vi "Fit VI window to Panel Center.vi"(4 "Error In":errorcluster, 6 "Panel Ref":refnum<vi>, 7 "VI Ref (calling VI)":refnum<vi>) -> (0 "Error Out":errorcluster, 3 "dup VI Ref":refnum<vi>)   [LabVIEW 2017]
doc: "This VI is designed to center a callee VI's window in a caller VI's window.\n\nAuthored by Brandon Steele\nsupport@mooregoodideas.com\nwww.mooregoodideas.com\n\nCopyright (c) 2010, Moore Good Ideas, Inc.\n\nAll rights reserved.\n\nRedistribution and use in source and binary forms, with or without modification, are permitted provided that the following conditions are met:\n\n * Redistributions of source code must retain the above copyright notice, this list of conditions and the following disclaimer.\n * Redistributions in binary form must reproduce the above copyright notice, this list of conditions and the following disclaimer in the documentation and/or other materials provided with the distribution.\n * Neither the name of Moore Good Ideas, Inc. nor the names of its contributors may be used to endorse or promote products derived from this software without specific prior written permission.\n\nTHIS SOFTWARE IS PROVIDED BY THE COPYRIGHT HOLDERS AND CONTRIBUTORS \"AS IS\" AND ANY EXPRESS OR IMPLIED WARRANTIES, INCLUDING, BUT NOT LIMITED TO, THE IMPLIED WARRANTIES OF MERCHANTABILITY AND FITNESS FOR A PARTICULAR PURPOSE ARE DISCLAIMED. IN NO EVENT SHALL THE COPYRIGHT OWNER OR CONTRIBUTORS BE LIABLE FOR ANY DIRECT, INDIRECT, INCIDENTAL, SPECIAL, EXEMPLARY, OR CONSEQUENTIAL DAMAGES (INCLUDING, BUT NOT LIMITED TO, PROCUREMENT OF SUBSTITUTE GOODS OR SERVICES; LOSS OF USE, DATA, OR PROFITS; OR BUSINESS INTERRUPTION) HOWEVER CAUSED AND ON ANY THEORY OF LIABILITY, WHETHER IN CONTRACT, STRICT LIABILITY, OR TORT (INCLUDING NEGLIGENCE OR OTHERWISE) ARISING IN ANY WAY OUT OF THE USE OF THIS SOFTWARE, EVEN IF ADVISED OF THE POSSIBILITY OF SUCH DAMAGE."
panel:
  in  "Pane Ref":refnum<vi>
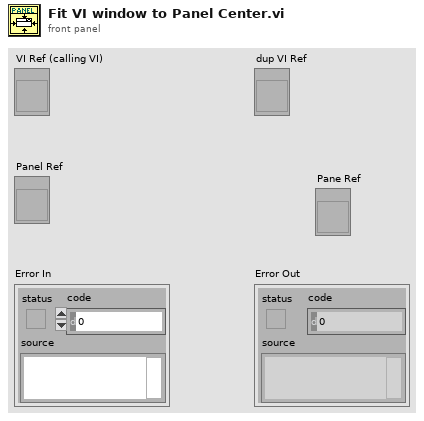
[diagram p1: front panel]
types:
  T1 = typedef "LVRectTypeDef.ctl" = cluster{"Left":i16, "Top":i16, "Right":i16, "Bottom":i16}
  T2 = cluster{"left":i16, "top":i16, "right":i16, "bottom":i16}
  T3 = typedef "LVAllMonitorsDisplayTypeDef.ctl" = cluster{"Bounds":cluster{"Left":i16, "Top":i16, "Right":i16, "Bottom":i16}, "Depth":i16}[]
  T4 = cluster{"Left":i16, "Top":i16, "Right":i16, "Bottom":i16}
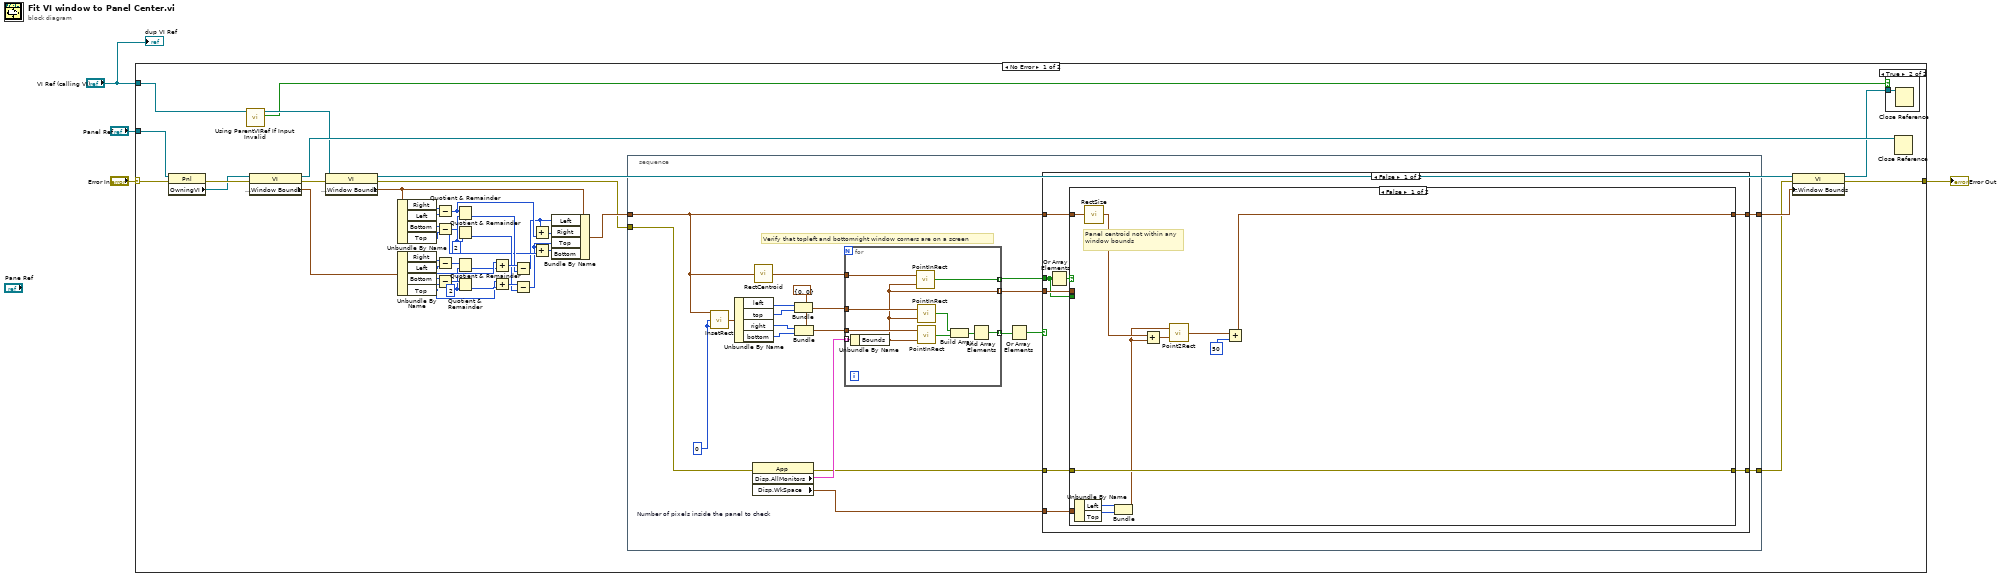
[diagram p0: block diagram]
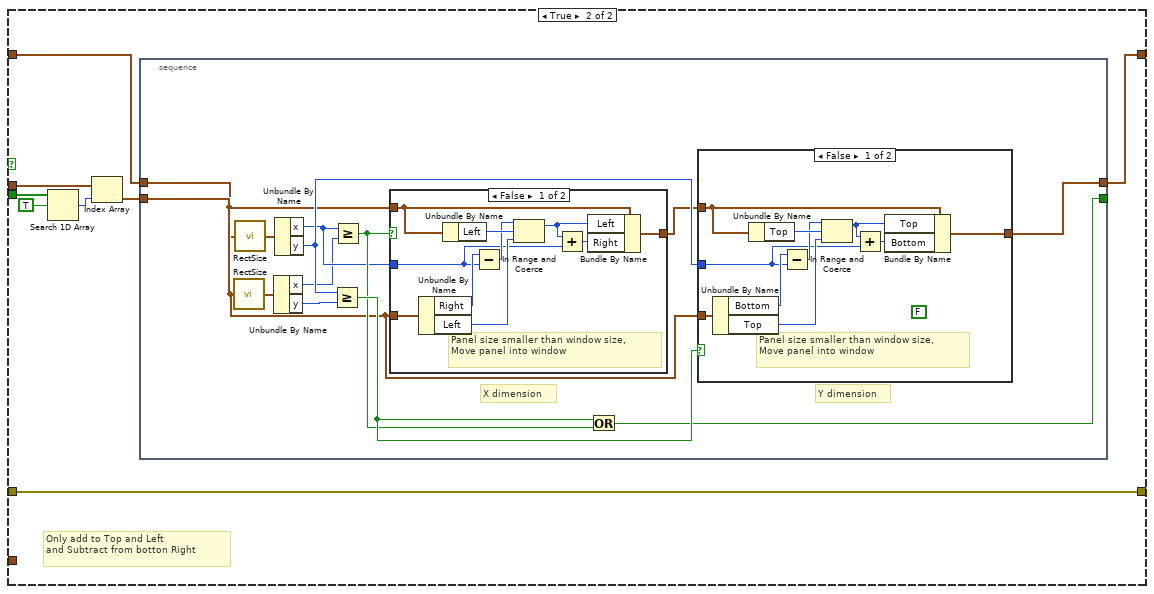
[diagram p2: hidden frame]
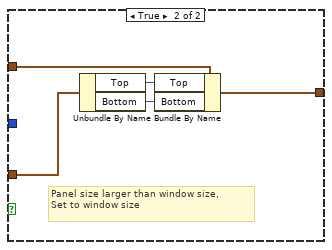
[diagram p3: hidden frame]
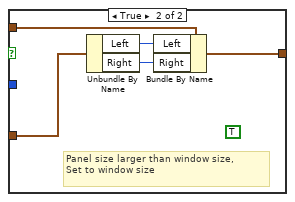
[diagram p4: hidden frame]
diagram:
  n1 = case shown="No Error" "Error In" {
    selector: "Error In" -> [w8 w151]
    tunnel: [w46 w151] -> w4
    tunnel: "Panel Ref" -> [w5 _]
    tunnel: "VI Ref (calling VI)" -> [w22 _]
    frame No Error {
      w39 = i16 2 ("y")
      w23 = i16 2 ("y")
      n2 = property class="Pnl"(reference=w5, error in=w8) -> (error out=w7:errorcluster, "OwningVI"=w6:refnum<vi>)  [unwired: 1 out]
      n3 = call "Using ParentVIRef If Input Invalid.vi"("VI Ref (calling VI)"=w22) -> ("Using Parent Ref(Need to Destroy)"=w11:bool, "VI Ref"=w19:refnum<vi>)  [unwired: 5 in]
      n4 = property class="VI"(reference=w6, error in=w7) -> (reference out=w21:refnum<vi>, error out=w40:errorcluster, "Front Panel Window:Window Bounds"=w45:T1)
      n5 = property class="VI"(reference=w19, error in=w40) -> (reference out=w26:refnum<vi>, error out=w10:errorcluster, "Front Panel Window:Window Bounds"=w14:T1)
      n6 = Unbundle By Name(w14) -> ("Right"=w35:i16, "Left"=w36:i16, "Bottom"=w37:i16, "Top"=w38:i16)
      n7 = Unbundle By Name(w45) -> ("Right"=w44:i16, "Left"=w34:i16, "Bottom"=w43:i16, "Top"=w31:i16)
      n8 = Subtract(x=w35, y=w36) -> (x-y=w25:i16)
      n9 = Subtract(x=w37, y=w38) -> (x-y=w24:i16)
      n10 = Subtract(x=w44, y=w34) -> (x-y=w42:i16)
      n11 = Subtract(x=w43, y=w31) -> (x-y=w41:i16)
      n12 = Quotient & Remainder(x=w25, y=w39) -> (floor(x/y)=w29:i16)  [unwired: 1 out]
      n13 = Quotient & Remainder(x=w24, y=w39) -> (floor(x/y)=w27:i16)  [unwired: 1 out]
      n14 = Quotient & Remainder(x=w42, y=w23) -> (floor(x/y)=w33:i16)  [unwired: 1 out]
      n15 = Quotient & Remainder(x=w41, y=w23) -> (floor(x/y)=w32:i16)  [unwired: 1 out]
      n16 = Add(x=w34, y=w33) -> (x+y=w30:i16)
      n17 = Add(x=w31, y=w32) -> (x+y=w28:i16)
      n18 = Subtract(x=w30, y=w29) -> (x-y=w17:i16)
      n19 = Subtract(x=w28, y=w27) -> (x-y=w16:i16)
      n20 = Add(x=w17, y=w25) -> (x+y=w15:i16)
      n21 = Add(x=w16, y=w24) -> (x+y=w18:i16)
      n22 = Bundle By Name(cluster=w14, "Left"=w17, "Right"=w15, "Top"=w16, "Bottom"=w18) -> (w13:T1)
      n23 = stacked-sequence {
        tunnel: [w57] -> w9
        tunnel: [w48] -> w12
        tunnel: w10 -> [w50]
        tunnel: w13 -> [w64]
        frame #0 {
          w59 = i16 0  # Number of pixels inside the panel to check
          w63 = cluster{"x":i16, "y":i16} {"x"=0, "y"=0} ("point")
          # "Verify that topleft and bottomright window corners are on a screen"
          n24 = call <vilib>:"InsetRect.vi"("dv"=w59, "dh"=w59, "rect"=w64) -> ("inset rect"=w53:T2)
          n25 = Unbundle By Name(w53) -> ("left"=w51:i16, "top"=w52:i16, "right"=w60:i16, "bottom"=w61:i16)
          n26 = property class="App"(error in=w50) -> (error out=w47:errorcluster, "Disp.AllMonitors"=w49:T3, "Disp.WkSpace"=w58:T1)  [unwired: 1 in, 1 out]
          n27 = call <vilib>:"RectCentroid.vi"("rect"=w64) -> ("point"=w65:cluster{"x":i16, "y":i16})
          n28 = Bundle(cluster=w63, "x"=w51, "y"=w52) -> (w54:cluster{"x":i16, "y":i16})
          n29 = Bundle(cluster=w63, "x"=w60, "y"=w61) -> (w62:cluster{"x":i16, "y":i16})
          n30 = for {
            tunnel: w49 -> [w149] mode=indexing
            tunnel: w54 -> [w148]
            tunnel: [w144] -> w55 mode=indexing
            tunnel: w62 -> [w143]
            tunnel: w65 -> [w142]
            tunnel: [w141] -> w66 mode=indexing
            tunnel: [w140] -> w67 mode=indexing
            n31 = Unbundle By Name(w149) -> ("Bounds"=w140:T4)
            n32 = call <vilib>:"PointInRect.vi"("rect"=w140, "point"=w142) -> ("pt in rect"=w141:bool)
            n33 = call <vilib>:"PointInRect.vi"("rect"=w140, "point"=w148) -> ("pt in rect"=w147:bool)
            n34 = call <vilib>:"PointInRect.vi"("rect"=w140, "point"=w143) -> ("pt in rect"=w146:bool)
            n35 = Build Array(w147, w146) -> (w145:bool[])
            n36 = And Array Elements(Boolean array=w145) -> (logical AND=w144:bool)
          }
          n37 = Or Array Elements(Boolean array=w55) -> (logical OR=w56:bool)
          n38 = case shown="False" w56 {
            tunnel: w47 -> [w70 w139]
            tunnel: [w69 w139] -> w57
            tunnel: w64 -> [w74 w138]
            tunnel: [w73 w138] -> w48
            tunnel: w58 -> [w75 _]
            tunnel: w66 -> [w68 _]
            tunnel: w67 -> [w71 _]
            frame False {
              n39 = Or Array Elements(Boolean array=w68) -> (logical OR=w72:bool)
              n40 = case shown="False" w72 {
                tunnel: w75 -> [w86 _]
                tunnel: w74 -> [w82 w89]
                tunnel: [w80 w87] -> w73
                tunnel: w71 -> [_ w91]
                tunnel: w70 -> [w79 w94]
                tunnel: [w79 w94] -> w69
                tunnel: w68 -> [_ w93]
                frame False {
                  # "Panel centroid not within any\nwindow bounds"
                  n41 = Unbundle By Name(w86) -> ("Left"=w85:i16, "Top"=w84:i16)
                  n42 = call <vilib>:"RectSize.vi"("rect"=w82) -> ("point"=w78:cluster{"x":i16, "y":i16})
                  n43 = Bundle("Left"=w85, "Top"=w84) -> (w76:cluster{"Left":i16, "Top":i16})  [unwired: 1 in]
                  n44 = Add(x=w78, y=w76) -> (x+y=w77:cluster{i16, i16})
                  n45 = call <vilib>:"Point2Rect.vi"("point b"=w77, "point a"=w76) -> ("rect"=w81:T2)
                  n46 = Add(x=w81, y=i16 50) -> (x+y=w80:T2)
                }
                frame True {
                  # "Only add to Top and Left\nand Subtract from botton Right"
                  n47 = Search 1D Array(1D array=w93, element=TRUE) -> (index of element=w90:i32)  [unwired: 1 in]
                  n48 = Index Array(array=w91, index=w90) -> (element=w88:T4)
                  n49 = stacked-sequence {
                    tunnel: [w95] -> _
                    tunnel: [w105] -> w87
                    tunnel: w88 -> [w104]
                    tunnel: w89 -> [w96]
                    frame #0 {
                      # "X dimension"
                      # "Y dimension"
                      n50 = call <vilib>:"RectSize.vi"("rect"=w104) -> ("point"=w98:cluster{"x":i16, "y":i16})
                      n51 = call <vilib>:"RectSize.vi"("rect"=w96) -> ("point"=w97:cluster{"x":i16, "y":i16})
                      n52 = Unbundle By Name(w98) -> ("x"=w99:i16, "y"=w102:i16)
                      n53 = Unbundle By Name(w97) -> ("x"=w100:i16, "y"=w103:i16)
                      n54 = Greater Or Equal?(x=w103, y=w102) -> (x >= y?=w107:bool)
                      n55 = Greater Or Equal?(x=w100, y=w99) -> (x >= y?=w106:bool)
                      n56 = case shown="False" w106 {
                        tunnel: w104 -> [w132 w133]
                        tunnel: w96 -> [w124 w134]
                        tunnel: w100 -> [w125 _]
                        tunnel: [w123 w135] -> w101
                        frame False {
                          # "Panel size smaller than window size,\nMove panel into window"
                          n57 = Unbundle By Name(w132) -> ("Right"=w128:i16, "Left"=w130:i16)
                          n58 = Unbundle By Name(w124) -> ("Left"=w131:i16)
                          n59 = Subtract(x=w128, y=w125) -> (x-y=w129:i16)
                          n60 = In Range and Coerce(upper limit=w129, x=w131, lower limit=w130) -> (coerced(x)=w127:i16)  [unwired: 1 out]
                          n61 = Add(x=w127, y=w125) -> (x+y=w126:i16)
                          n62 = Bundle By Name(cluster=w124, "Left"=w127, "Right"=w126) -> (w123:T1)
                        }
                        frame True {
                          (unwired) TRUE
                          # "Panel size larger than window size,\nSet to window size"
                          n63 = Unbundle By Name(w133) -> ("Left"=w137:i16, "Right"=w136:i16)
                          n64 = Bundle By Name(cluster=w134, "Left"=w137, "Right"=w136) -> (w135:T1)
                        }
                      }
                      n65 = Or(x=w107, y=w106) -> (x .or. y?=w95:bool)
                      n66 = case shown="False" w107 {
                        tunnel: w104 -> [w117 w122]
                        tunnel: w101 -> [w109 w118]
                        tunnel: w103 -> [w110 _]
                        tunnel: [w108 w119] -> w105
                        frame False {
                          (unwired) FALSE
                          # "Panel size smaller than window size,\nMove panel into window"
                          n67 = Unbundle By Name(w117) -> ("Bottom"=w113:i16, "Top"=w115:i16)
                          n68 = Unbundle By Name(w109) -> ("Top"=w116:i16)
                          n69 = Subtract(x=w113, y=w110) -> (x-y=w114:i16)
                          n70 = In Range and Coerce(upper limit=w114, x=w116, lower limit=w115) -> (coerced(x)=w112:i16)  [unwired: 1 out]
                          n71 = Add(x=w112, y=w110) -> (x+y=w111:i16)
                          n72 = Bundle By Name(cluster=w109, "Top"=w112, "Bottom"=w111) -> (w108:T1)
                        }
                        frame True {
                          # "Panel size larger than window size,\nSet to window size"
                          n73 = Unbundle By Name(w122) -> ("Top"=w121:i16, "Bottom"=w120:i16)
                          n74 = Bundle By Name(cluster=w118, "Top"=w121, "Bottom"=w120) -> (w119:T1)
                        }
                      }
                    }
                  }
                }
              }
            }
            frame True {
            }
          }
        }
      }
      n75 = property class="VI"(reference=w26, error in=w9, "Front Panel Window:Window Bounds"=w12) -> (reference out=w20:refnum<vi>, error out=w46:errorcluster)
      n76 = case shown="True" w11 {
        tunnel: w20 -> [_ w150]
        frame False {
        }
        frame True {
          n77 = Close Reference(reference=w150) -> ()  [unwired: 1 in, 1 out]
        }
      }
      n78 = Close Reference(reference=w21) -> ()  [unwired: 1 in, 1 out]
    }
    frame Error {
    }
  }
  "Error Out" <- w4
  "dup VI Ref" <- "VI Ref (calling VI)"
